vi "P.80 2019.1.16.vi"() -> ()   [LabVIEW 2010]
uses:
  <vilib>/DAQmx/read.llb/DAQmx Read (Analog DBL 1Chan 1Samp).vi
  <vilib>/DAQmx/write.llb/DAQmx Write (Analog DBL 1Chan 1Samp).vi
  <vilib>/DAQmx/create/channels.llb/DAQmx Create Channel (AI-Voltage-Basic).vi
  <vilib>/DAQmx/configure/timing.llb/DAQmx Timing (Sample Clock).vi
  <vilib>/DAQmx/create/channels.llb/DAQmx Create Channel (AO-Voltage-Basic).vi
  <vilib>/measure/maspectr.llb/FFT Spectrum (Mag-Phase) for 1 Chan.vi
  <vilib>/daqmx/miscellaneous.llb/DAQmx Fill In Error Info.vi
  <vilib>/measure/NI_MAPro.lvlib
panel:
  out "Waveform Graph":cluster{"f0":dbl, "df":dbl, "magnitude":dbl[]}(graph)
  out "模擬輸入x(t) 2":dbl(graph)
  out "理想迴圈時間":dbl
  out "延遲警告":bool
  in  "DAQ input":tag
  in  "DAQ output":tag
  out "message":string=" INSTRUCTIONS:\r\rNormal Use:  When using subVIs that incorporate the error in/error out (or error I/O) structure, place this handler where you want to inform the user of an error, typically at the end of the I/O data path, as the last action of the program.  If the error in error? is ERROR, the handler creates a message describing the error and its source.  If the type of dialog = 1 (default), the message is displayed to the user, who can only acknowedge it.  If the type = 2, the user can acknowledge the message or abort execution; aborting a program with active I/O is not recommended.  If the type = 0, no message is displayed; this is used to process the error programmatically, and the error out cluster elements are wired to individual terminals for that reason.  \r\rOther Use:\n\r\nlocal testing.  To test the error code of a subVI or function that does not have the error I/O structure, you can wire its error code and a source string to the local error code and error source inputs.  If error in error? indicates no error and error code is not equal to 0, the local code and source are substituted for the error in values, and error? is set TRUE (ERROR)."
  out "while平均運行時間":dbl
  in  "取樣頻率":dbl=9000.0 min=1.0 max=20000.0 step=1.0
  in  "stop":bool
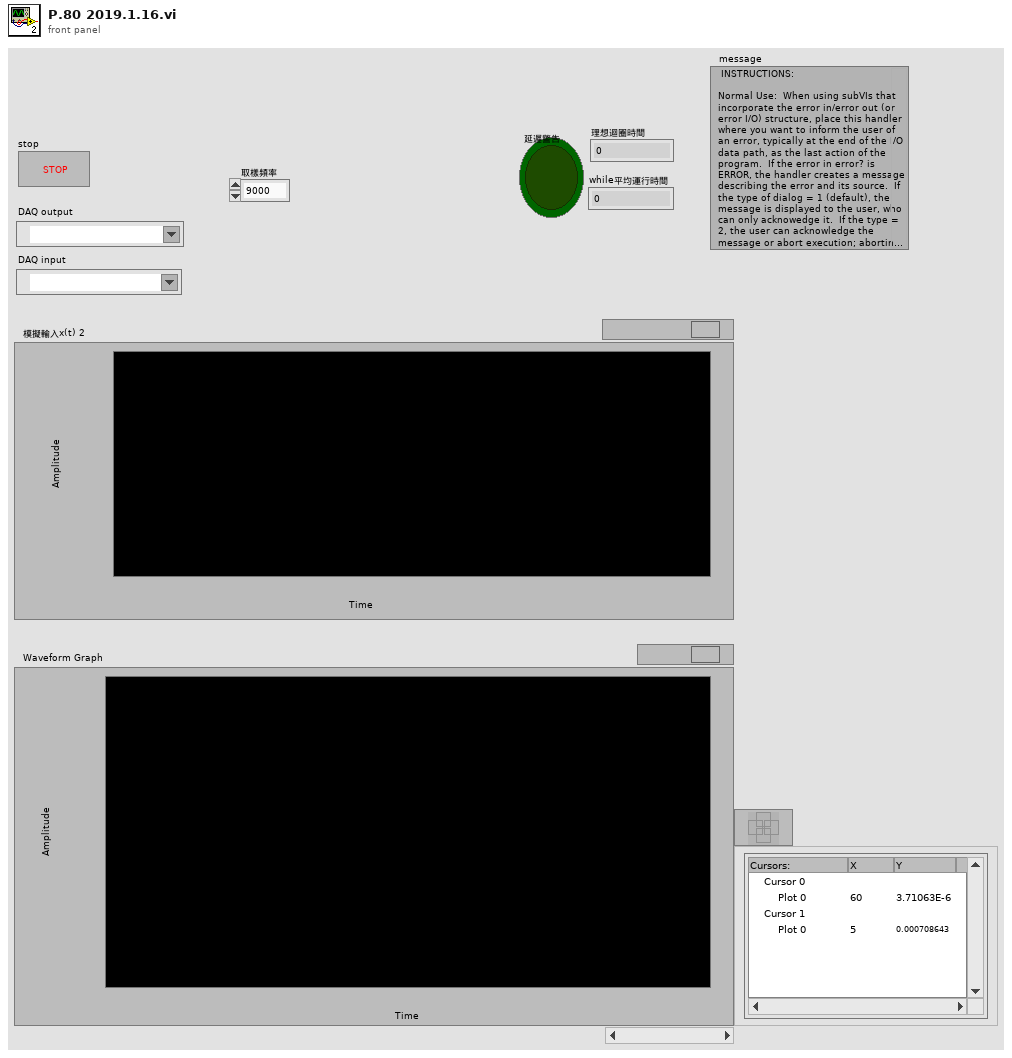
[diagram p1: front panel]
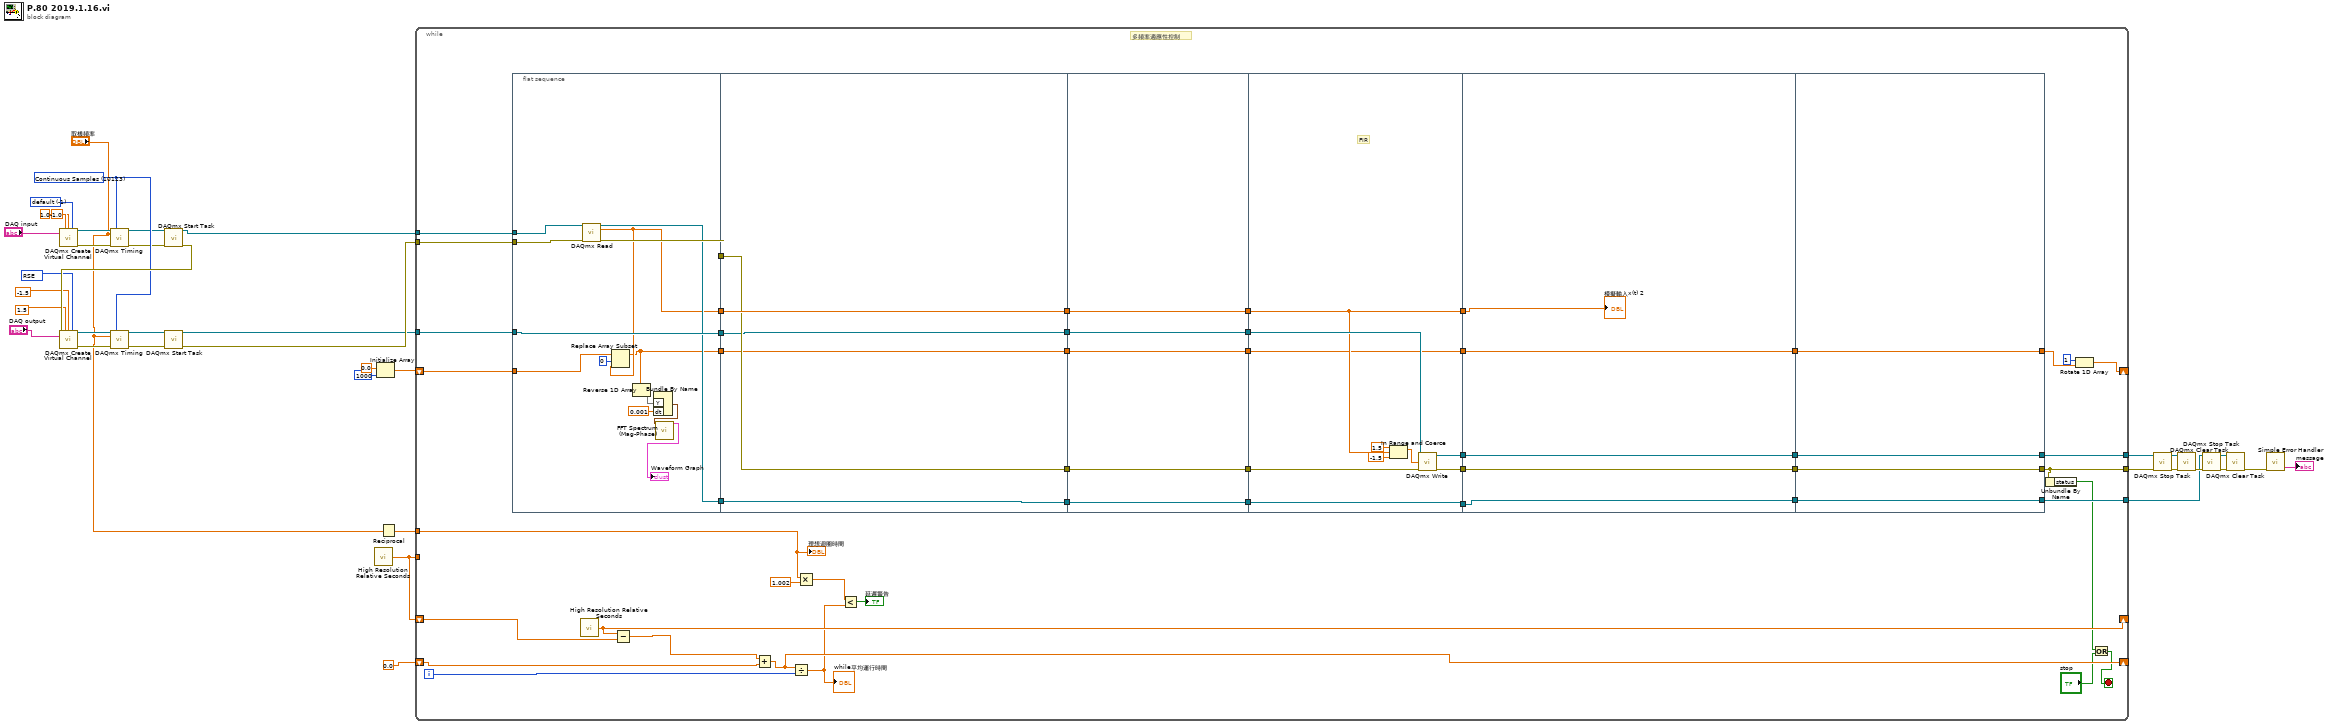
[diagram p0: block diagram]
diagram:
  w32 = 10123 items=["Finite Samples"=10178, "Continuous Samples"=10123, "Hardware Timed Single Point"=12522] ("sample mode")
  w29 = 10083 items=["Default"=-1, "RSE"=10083, "Differential"=10106, "Pseudodifferential"=12529] ("output terminal configuration")
  w28 = -1 items=["default"=-1, "RSE"=10083, "NRSE"=10078, "Differential"=10106, "Pseudodifferential"=12529] ("input terminal configuration")
  n1 = call-poly <vilib>:"DAQmx Create Virtual Channel.vi"("maximum value"=1.0, "minimum value"=-1.0, "input terminal configuration"=w28, "physical channels"="DAQ input") -> ("task out"=w20:refnum<k21>, "error out"=w23:errorcluster)  [unwired: 10 in]
  n2 = call-poly <vilib>:"DAQmx Timing.vi"("task/channels in"=w20, "sample mode"=w32, "rate"="取樣頻率", "error in"=w23) -> ("task out"=w21:refnum<k21>, "error out"=w22:errorcluster)  [unwired: 10 in]
  n3 = call <vilib>:"DAQmx Start Task.vi"("task/channels in"=w21, "error in"=w22) -> ("task out"=w19:refnum<k21>, "error out"=w35:errorcluster)  [unwired: 12 in]
  n4 = call-poly <vilib>:"DAQmx Create Virtual Channel.vi"("maximum value"=1.5, "minimum value"=-1.5, "output terminal configuration"=w29, "physical channels"="DAQ output", "error in"=w35) -> ("task out"=w27:refnum<k21>, "error out"=w24:errorcluster)  [unwired: 9 in]
  n5 = call-poly <vilib>:"DAQmx Timing.vi"("task/channels in"=w27, "sample mode"=w32, "rate"="取樣頻率", "error in"=w24) -> ("task out"=w26:refnum<k21>, "error out"=w25:errorcluster)  [unwired: 10 in]
  n6 = call <vilib>:"DAQmx Start Task.vi"("task/channels in"=w26, "error in"=w25) -> ("task out"=w17:refnum<k21>, "error out"=w18:errorcluster)  [unwired: 12 in]
  n7 = call <vilib>:"High Resolution Relative Seconds.vi"() -> ("relative seconds"=w38:dbl)
  n8 = Initialize Array(0.0 ("element"), 1000 ("dimension size")) -> (w3:dbl[])
  n9 = Reciprocal(x="取樣頻率") -> (1/x=w4:dbl)
  n10 = while {
    tunnel: w38 -> [_]
    shift-right: [w83] -> _
    shift-left: w38 -> [w82]
    shift-right: [w84] -> _
    shift-left: 0.0 -> [w86]
    tunnel: w19 -> [w78]
    tunnel: w18 -> [w77]
    tunnel: w17 -> [w76]
    tunnel: [w72] -> w11
    tunnel: [w63] -> w10
    tunnel: [w66] -> w9
    tunnel: w4 -> [w52]
    shift-right: [w40] -> _
    shift-left: w3 -> [w47]
    i -> [w85]
    stop <- w65 stop-if-true
    # "多頻率適應性控制"
    n11 = flat-sequence {
      tunnel: [w93] -> w80
      tunnel: [w97] -> w79
      tunnel: w78 -> [w99]
      tunnel: w77 -> [w98]
      tunnel: w76 -> [w96]
      tunnel: [w96] -> w75
      tunnel: [w95] -> w69
      tunnel: w47 -> [w94]
      tunnel: [w91] -> w42
      tunnel: [w103] -> w61
      tunnel: [w104] -> w59
      tunnel: w80 -> [w104]
      tunnel: w79 -> [w103]
      tunnel: [w102] -> w57
      tunnel: w75 -> [w102]
      tunnel: [w101] -> w55
      tunnel: w69 -> [w101]
      tunnel: [w100] -> w43
      tunnel: w42 -> [w100]
      tunnel: w61 -> [w109]
      tunnel: [w109] -> w60
      tunnel: w59 -> [w108]
      tunnel: [w108] -> w58
      tunnel: w57 -> [w107]
      tunnel: [w107] -> w56
      tunnel: w55 -> [w106]
      tunnel: [w106] -> w54
      tunnel: [w105] -> w44
      tunnel: w43 -> [w105]
      tunnel: w60 -> [w118]
      tunnel: [w111] -> w81
      tunnel: w58 -> [w111]
      tunnel: w56 -> [w119]
      tunnel: [w117] -> w73
      tunnel: [w116] -> w71
      tunnel: w54 -> [w115]
      tunnel: [w115] -> w68
      tunnel: [w110] -> w45
      tunnel: w44 -> [w110]
      tunnel: w81 -> [w121]
      tunnel: [w124] -> w74
      tunnel: w73 -> [w124]
      tunnel: w71 -> [w123]
      tunnel: [w123] -> w70
      tunnel: w68 -> [w122]
      tunnel: [w122] -> w67
      tunnel: [w120] -> w46
      tunnel: w45 -> [w120]
      tunnel: w74 -> [w128]
      tunnel: [w128] -> w72
      tunnel: [w127] -> w63
      tunnel: w70 -> [w127]
      tunnel: w67 -> [w126]
      tunnel: [w126] -> w66
      tunnel: [w125] -> w41
      tunnel: w46 -> [w125]
      frame #0 {
        n12 = call-poly <vilib>:"DAQmx Read.vi"("task/channels in"=w99, "error in"=w98) -> ("task out"=w95:refnum<k21>, "data"=w93:dbl, "error out"=w97:errorcluster)  [unwired: 11 in]
        n13 = Replace Array Subset(array=w94, new element=w93, index=0) -> (w91:dbl[])
        n14 = Reverse 1D Array(array=w91) -> (reversed array=w89:dbl[])
        n15 = Bundle By Name("Y"=w89, "dt"=0.001) -> (w90:waveform(dbl))  [unwired: 1 in]
        n16 = call-poly <vilib>:"FFT Spectrum (Mag-Phase).vi"("time signal"=w90) -> ("magnitude"=→"Waveform Graph":cluster{"f0":dbl, "df":dbl, "magnitude":dbl[]})  [unwired: 6 in, 4 out]
      }
      frame #1 {
      }
      frame #2 {
      }
      frame #3 {
        # "FIR"
        n17 = In Range and Coerce(upper limit=1.5, x=w111, lower limit=-1.5) -> (coerced(x)=w114:dbl)  [unwired: 1 out]
        n18 = call-poly <vilib>:"DAQmx Write.vi"("task/channels in"=w119, "data"=w114, "error in"=w118) -> ("task out"=w117:refnum<k21>, "error out"=w116:errorcluster)  [unwired: 10 in, 1 out]
      }
      frame #4 {
        "模擬輸入x(t) 2" <- w121
      }
      frame #5 {
      }
    }
    n19 = call <vilib>:"High Resolution Relative Seconds.vi"() -> ("relative seconds"=w83:dbl)
    n20 = Subtract(x=w83, y=w82) -> (x-y=w53:dbl)
    n21 = Add(x=w53, y=w86) -> (x+y=w84:dbl)
    n22 = Divide(x=w84, y=w85) -> (x/y=w49:dbl)
    "while平均運行時間" <- w49
    n23 = Multiply(x=w52, y=1.002) -> (x*y=w50:dbl)
    n24 = Less?(x=w50, y=w49) -> (x < y?=→"延遲警告":bool)
    n25 = Unbundle By Name(w63) -> ("status"=w62:bool)
    n26 = Rotate 1D Array(1:w41, 2:1 ("n")) -> (0:w40:dbl[])
    n27 = Or(x=w62, y="stop") -> (x .or. y?=w65:bool)
    "理想迴圈時間" <- w52
  }
  n28 = call <vilib>:"DAQmx Stop Task.vi"("task/channels in"=w11, "error in"=w10) -> ("task out"=w12:refnum<k21>, "error out"=w13:errorcluster)  [unwired: 12 in]
  n29 = call <vilib>:"DAQmx Clear Task.vi"("task in"=w12, "error in"=w13) -> ("error out"=w16:errorcluster)  [unwired: 13 in]
  n30 = call <vilib>:"DAQmx Stop Task.vi"("task/channels in"=w9, "error in"=w16) -> ("task out"=w15:refnum<k21>, "error out"=w14:errorcluster)  [unwired: 12 in]
  n31 = call <vilib>:"DAQmx Clear Task.vi"("task in"=w15, "error in"=w14) -> ("error out"=w8:errorcluster)  [unwired: 13 in]
  n32 = call <vilib>:"Simple Error Handler.vi"("error in (no error)"=w8) -> ("message"=→"message":string)  [unwired: 4 in, 4 out]
